vi "Generate header file.vi"(8 "error in (no error)":errorcluster, 9 "Pixmap":u16[][](array[numeric]) format="%x", 10 "folder to output file":path, 11 "path to image file (png, jpeg, jpg, bmp)":path) -> (0 "error out":errorcluster)   [LabVIEW 2019, in "LabVIEW RGB565 Convertor.lvlib"]
uses:
  LabVIEW RGB565 Convertor.lvlib
  def-header file template.ctl
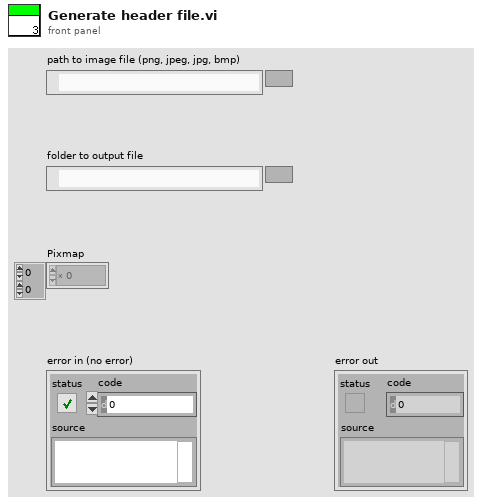
[diagram p1: front panel]
types:
  T1 = enum16{"open", "replace", "create", "open or create", "replace or create", "replace or create with confirmation"}
  T2 = typedef "LabVIEW RGB565 Convertor.lvlib/def-header file template.ctl" = cluster{"HeaderFileDefine":string, "GeneratedFrom":string, "TimeGenerated":string, "ImageSize":string, "ImageName":string, "PixNumber":string, "PixMap":string}
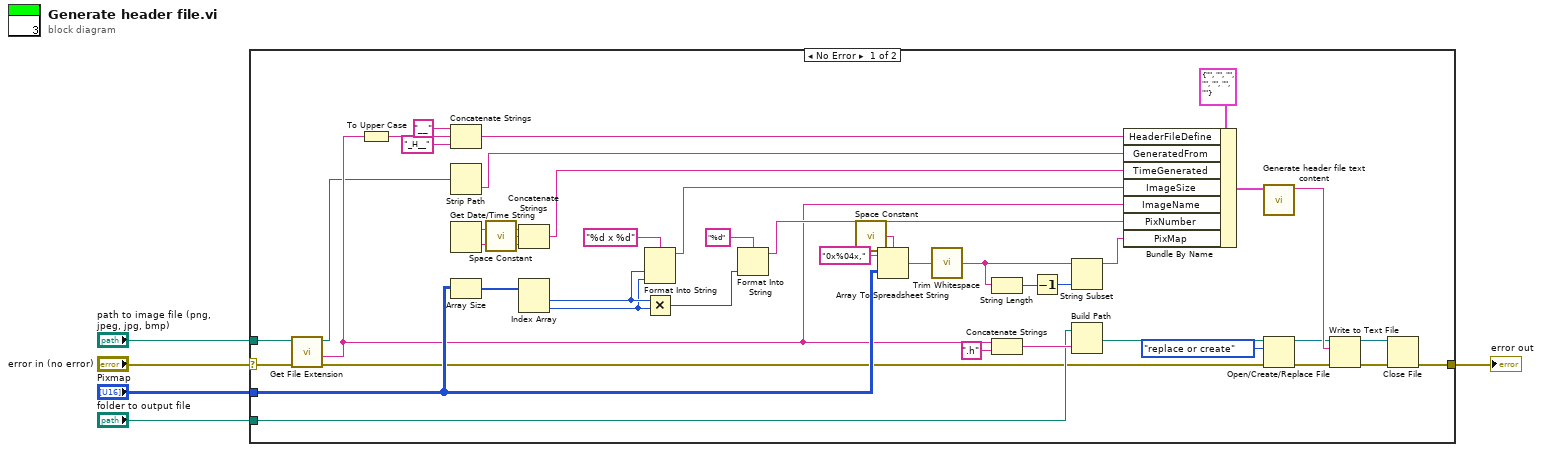
[diagram p0: block diagram]
diagram:
  n1 = case shown="No Error" "error in (no error)" {
    selector: "error in (no error)" -> [w38 w49]
    tunnel: "Pixmap" -> [w40 _]
    tunnel: "path to image file (png, jpeg, jpg, bmp)" -> [w30 _]
    tunnel: [w24 w49] -> w3
    tunnel: "folder to output file" -> [w29 _]
    frame No Error {
      n2 = call <vilib>:"Get File Extension.vi"("error in (no error)"=w38, "file"=w30) -> ("error out"=w21:errorcluster, "filename without extension"=w17:string, "dup file"=w13:path)  [unwired: 5 in, 2 out]
      n3 = To Upper Case(1:w17) -> (0:w15:string)
      n4 = Concatenate Strings("__" ("string"), w15, "_H__" ("string")) -> (w16:string)
      n5 = Strip Path(path=w13) -> (name=w31:string)  [unwired: 1 out]
      n6 = Get Date/Time String() -> (date string=w48:string, time string=w47:string)  [unwired: 3 in]
      n7 = Array Size(array=w40) -> (size(s)=w44:i32[])
      n8 = call <vilib>:"Space Constant.vi"() -> ("String"=w46:string)
      n9 = Concatenate Strings(w48, w46, w47) -> (w34:string)
      n10 = Index Array(array=w44) -> (element #1=w42:i32, element #2=w41:i32)  [unwired: 2 in]
      n11 = Format Into String(format string="%d x %d", w42, w41) -> (resulting string=w18:string)  [unwired: 2 in, 1 out]
      n12 = Multiply(x=w42, y=w41) -> (x*y=w10:i32)
      n13 = Format Into String(format string="%d", w10) -> (resulting string=w33:string)  [unwired: 2 in, 1 out]
      n14 = call <vilib>:"Space Constant.vi"() -> ("String"=w11:string)
      n15 = Array To Spreadsheet String(delimiter (Tab)=w11, array=w40, 3:"0x%04x," ("format string")) -> (spreadsheet string=w25:string)
      n16 = call <vilib>:"Trim Whitespace.vi"("string"=w25) -> ("trimmed string"=w7:string)  [unwired: 1 in]
      n17 = String Length(string=w7) -> (length=w8:i32)
      n18 = Concatenate Strings(w17, ".h" ("string")) -> (w37:string)
      n19 = Decrement(x=w8) -> (x-1=w6:i32)
      n20 = String Subset(string=w7, length (rest)=w6) -> (substring=w9:string)  [unwired: 1 in]
      n21 = Build Path(base path=w29, name or relative path=w37) -> (appended path=w28:path)
      n22 = Bundle By Name(cluster=T2 {"HeaderFileDefine"="", "GeneratedFrom"="", "TimeGenerated"="", "ImageSize"="", "ImageName"="", "PixNumber"="", "PixMap"=""} ("header file template"), "HeaderFileDefine"=w16, "GeneratedFrom"=w31, "TimeGenerated"=w34, "ImageSize"=w18, "ImageName"=w17, "PixNumber"=w33, "PixMap"=w9) -> (w32:T2)
      n23 = call "Generate header file text content.vi"("header file template"=w32) -> ("header file content"=w27:string)  [unwired: 10 in]
      n24 = Open/Create/Replace File(file path (use dialog)=w28, error in=w21, operation (0:open)=T1."replace or create") -> (refnum out=w22:refnum<file>, error out=w20:errorcluster)  [unwired: 3 in, 1 out]
      n25 = Write to Text File(file (use dialog)=w22, text=w27, error in=w20) -> (refnum out=w23:refnum<file>, error out=w26:errorcluster)  [unwired: 1 in, 1 out]
      n26 = Close File(refnum=w23, error in=w26) -> (error out=w24:errorcluster)  [unwired: 1 out]
    }
    frame Error {
    }
  }
  "error out" <- w3
